vi "Write strings to Spreadsheet.vi"(1 "transpose? (no:F)":bool, 4 "format (%s)":string="%s", 5 "append to file? (new file:F)":bool, 6 "1D data":string[](array[string]), 7 "2D data":string[][](array[string]), 8 "file path (dialog if empty)":path) -> (3 "new file path (Not A Path if cancelled)":path)   [LabVIEW 2010]
doc: "Converts a 2D or 1D array of single-precision numbers to a text string and writes the string to a new byte stream file or appends the string to an existing file. You can optionally transpose the data. This VI opens or creates the file beforehand and closes it afterwards. You can use this VI to create a text file readable by most spreadsheet applications.\n\nfile path is the path name of the file. If file path is empty (default value) or is Not A Path, the VI displays a File dialog box from which you can select a file. Error 43 occurs if the user cancels the dialog. \n\n2D data contains the single-precision numbers the VI writes to the file if 1D data is not wired or is empty.\n\n1D data contains the single-precision numbers the VI writes to the file if this input is not empty. The VI converts the 1D array into a 2D array before transposing it and converting it to a string and writing it to the file. If transpose? is FALSE, each call to this VI creates a new line or row in the file.\n\nappend to file? Set to TRUE if you want to append the data to a existing file; you can also set it TRUE to write to a new file. Set to FALSE (default value) if you want to write the data to a new file or to replace an existing file. \n\ntranspose? Set TRUE to transpose the data before converting it to a string. The default value is FALSE.\n\nformat specifies how to convert the numbers to characters. If the format string is %.3f (default), the VI creates a string long enough to contain the number, with three digits to the right of the decimal point. If the format is %d, the VI converts the data to integer form using as many characters as necessary to contain the entire number. Refer to the discussion of format strings and the Array To Spreadsheet String function in Chapter 6, String Functions, of the LabVIEW Function Reference Manual.\n\nnew file path is the path of the file to which the VI wrote data. You can use this output to determine the path of a file that you open using dialog. new file path returns Not A Path if the user selects Cancel from the dialog box."
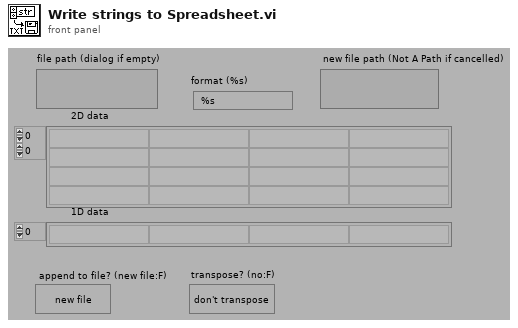
[diagram p1: front panel]
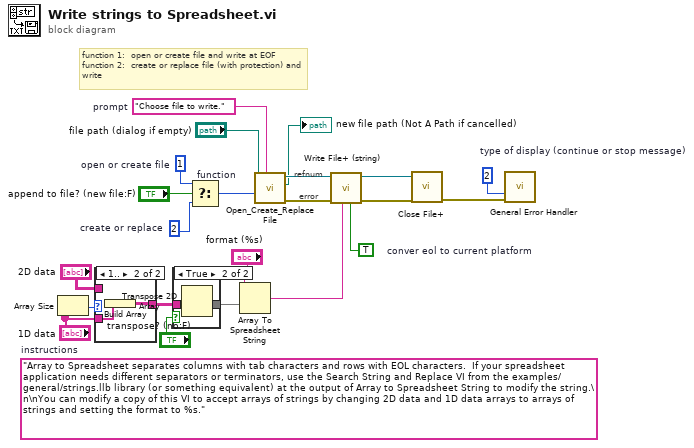
[diagram p0: block diagram]
diagram:
  (unwired) "Array to Spreadsheet separates columns with tab characters and rows with EOL characters.  If your spreadsheet application needs different separators or terminators, use the Search String and Replace VI from the examples/general/strings.llb library (or something equivalent) at the output of Array to Spreadsheet String to modify the string.\n\nYou can modify a copy of this VI to accept arrays of strings by changing 2D data and 1D data arrays to arrays of strings and setting the format to %s."  # instructions
  w1 = i16 2  # create or replace
  w4 = TRUE  # conver eol to current platform
  w20 = 2  # type of display (continue or stop message)
  w9 = "Choose file to write."  # prompt
  w21 = i16 1  # open or create file
  # "error"
  # "refnum"
  # "function 1:  open or create file and write at EOF\nfunction 2:  create or replace file (with protection) and write"
  n1 = Array Size(array="1D data") -> (size(s)=w18:i32)
  n2 = case shown="1.." w18 {
    tunnel: "1D data" -> [_ w25]
    tunnel: [w23 w24] -> w14
    tunnel: "2D data" -> [w23 _]
    frame ..0 {
      # "1D array is empty"
    }
    frame 1.. {
      n3 = Build Array(w25) -> (w24:string[][])
    }
  }
  n4 = case shown="True" "transpose? (no:F)" {
    tunnel: [w26 w28] -> w12
    tunnel: w14 -> [w26 w27]
    frame False {
    }
    frame True {
      n5 = Transpose 2D Array(2D array=w27) -> (transposed array=w28:string[][])
    }
  }
  n6 = Select "function"(t=w21, s="append to file? (new file:F)", f=w1) -> (s? t:f=w11:i16)
  n7 = Array To Spreadsheet String(array=w12, 3:"format (%s)") -> (spreadsheet string=w7:string)  [unwired: 1 in]
  n8 = call <vilib>:"Open_Create_Replace File.vi"("prompt"=w9, "function (open:0)"=w11, "file path"="file path (dialog if empty)") -> ("error out"=w8:errorcluster, "new file path"=→"new file path (Not A Path if cancelled)":path, "refnum"=w3:refnum<file>)  [unwired: 5 in, 1 out]
  n9 = call <vilib>:"Write File+ (string).vi"("convert eol? (no:F)"=w4, "string"=w7, "error in (no error)"=w8, "refnum"=w3) -> ("error out"=w19:errorcluster, "dup refnum"=w6:refnum<file>)  [unwired: 3 in, 1 out]
  n10 = call <vilib>:"Close File+.vi"("error in (no error)"=w19, "refnum"=w6) -> ("error out"=w5:errorcluster)  [unwired: 3 in, 2 out]
  n11 = call <vilib>:"General Error Handler.vi"("type of dialog (OK msg:1)"=w20, "error in (no error)"=w5) -> ()  [unwired: 9 in, 5 out]
